vi "Read Time.vi"(11 "Teller in":refnum<class "Teller.lvclass">) -> (2 "Time":timestamp)   [LabVIEW 2025, in "jettl.lvlib" / "Teller.lvlib" / "Teller.lvclass"]
uses:
  Teller.lvclass
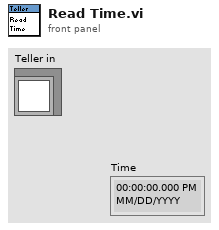
[diagram p1: front panel]
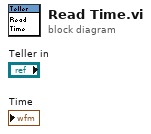
[diagram p0: block diagram]
diagram:
